vi "Globals.vi"() -> ()   [LabVIEW 2017, in "nifxpmath_IntAccumulator.xnode"]
uses:
  <vilib>/rvi/FXPMathLib/basic elements/FxpIntAccumulator/XNode/nifxpmath_IntAccumulator.xnode
panel:
  in  "Feedback scaling limit":u32=64
  in  "Term OVFL NAME":string="overflow"
  in  "Term EN NAME":string="enable (T)"
  in  "Term COUTNBOUT NAME":string="carry-out/inverted borrow-out"
  in  "Term CINNBIN NAME":string="carry-in/inverted borrow-in (F)"
  in  "Term ISSUB NAME":string="is sub? (F)"
  in  "Term LOAD NAME":string="load (F)"
  in  "Term S NAME":string="s"
  in  "Term X NAME":string="x"
  in  "Term EN ID":string="TERM_EN"
  in  "Term CINNBIN ID":string="TERM_CINNBIN"
  in  "Term COUTNBOUT ID":string="TERM_COUTNBOUT"
  in  "Term ISSUB ID":string="TERM_ISSUB"
  in  "Term LOAD ID":string="TERM_LOAD"
  in  "Term S ID":string="TERM_S"
  in  "Term X ID":string="TERM_X"
  out "SmallIcon":picture
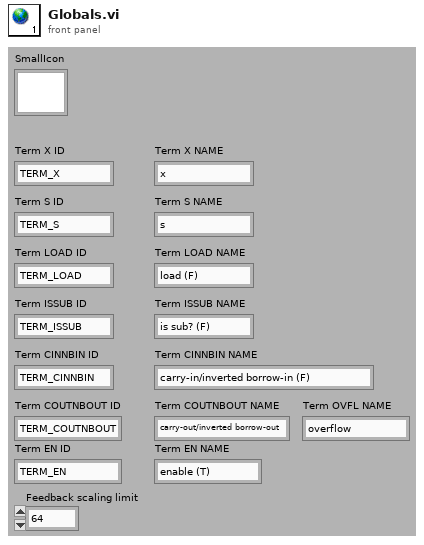
[diagram p1: front panel]
diagram:
